vi "read Txt Files.vi"(10 "file path (use dialog)":path) -> (1 "error out":errorcluster, 2 "number":T1)   [LabVIEW 2017] (continued)
0.000000\tVoltage¡G\t4.590790\nReal Periold(ms)¡G\t1\tEncoder Position(0.1mm)¡G\t1.000000\tVelocity(0.1mm0/s)¡G\t1000.000000\tVoltage¡G\t4.606384\nReal Periold(ms)¡G\t1\tEncoder Position(0.1mm)¡G\t3.000000\tVelocity(0.1mm0/s)¡G\t2000.000000\tVoltage¡G\t4.604797\nReal Periold(ms)¡G\t1\tEncoder Position(0.1mm)¡G\t11.000000\tVelocity(0.1mm0/s)¡G\t8000.000000\tVoltage¡G\t4.602234\nReal Periold(ms)¡G\t1\tEncoder Position(0.1mm)¡G\t25.000000\tVelocity(0.1mm0/s)¡G\t14000.000000\tVoltage¡G\t4.613708\nReal Periold(ms)¡G\t1\tEncoder Position(0.1mm)¡G\t47.000000\tVelocity(0.1mm0/s)¡G\t22000.000000\tVoltage¡G\t4.615601\nReal Periold(ms)¡G\t1\tEncoder Position(0.1mm)¡G\t83.000000\tVelocity(0.1mm0/s)¡G\t36000.000000\tVoltage¡G\t4.616241\nReal Periold(ms)¡G\t1\tEncoder Position(0.1mm)¡G\t119.000000\tVelocity(0.1mm0/s)¡G\t36000.000000\tVoltage¡G\t4.597778\nReal Periold(ms)¡G\t1\tEncoder Position(0.1mm)¡G\t165.000000\tVelocity(0.1mm0/s)¡G\t46000.000000\tVoltage¡G\t4.604462\nReal Periold(ms)¡G\t1\tEncoder Position(0.1mm)¡G\t217.000000\tVelocity(0.1mm0/s)¡G\t52000.000000\tVoltage¡G\t4.609253\nReal Periold(ms)¡G\t1\tEncoder Position(0.1mm)¡G\t272.000000\tVelocity(0.1mm0/s)¡G\t55000.000000\tVoltage¡G\t4.602570\nReal Periold(ms)¡G\t1\tEncoder Position(0.1mm)¡G\t332.000000\tVelocity(0.1mm0/s)¡G\t60000.000000\tVoltage¡G\t4.608612\nReal Periold(ms)¡G\t1\tEncoder Position(0.1mm)¡G\t392.000000\tVelocity(0.1mm0/s)¡G\t60000.000000\tVoltage¡G\t4.596497\nReal Periold(ms)¡G\t1\tEncoder Position(0.1mm)¡G\t454.000000\tVelocity(0.1mm0/s)¡G\t62000.000000\tVoltage¡G\t4.605408\nReal Periold(ms)¡G\t1\tEncoder Position(0.1mm)¡G\t517.000000\tVelocity(0.1mm0/s)¡G\t63000.000000\tVoltage¡G\t4.608276\nReal Periold(ms)¡G\t1\tEncoder Position(0.1mm)¡G\t580.000000\tVelocity(0.1mm0/s)¡G\t63000.000000\tVoltage¡G\t4.619110\nReal Periold(ms)¡G\t1\tEncoder Position(0.1mm)¡G\t645.000000\tVelocity(0.1mm0/s)¡G\t65000.000000\tVoltage¡G\t4.622284\nReal Periold(ms)¡G\t1\tEncoder Position(0.1mm)¡G\t713.000000\tVelocity(0.1mm0/s)¡G\t68000.000000\tVoltage¡G\t4.615295\nReal Periold(ms)¡G\t1\tEncoder Position(0.1mm)¡G\t777.000000\tVelocity(0.1mm0/s)¡G\t64000.000000\tVoltage¡G\t4.594604\nReal Periold(ms)¡G\t1\tEncoder Position(0.1mm)¡G\t841.000000\tVelocity(0.1mm0/s)¡G\t64000.000000\tVoltage¡G\t4.611481\nReal Periold(ms)¡G\t1\tEncoder Position(0.1mm)¡G\t907.000000\tVelocity(0.1mm0/s)¡G\t66000.000000\tVoltage¡G\t4.625153\nReal Periold(ms)¡G\t1\tEncoder Position(0.1mm)¡G\t976.000000\tVelocity(0.1mm0/s)¡G\t69000.000000\tVoltage¡G\t4.610840\nReal Periold(ms)¡G\t1\tEncoder Position(0.1mm)¡G\t1038.000000\tVelocity(0.1mm0/s)¡G\t62000.000000\tVoltage¡G\t4.601929\nReal Periold(ms)¡G\t1\tEncoder Position(0.1mm)¡G\t1105.000000\tVelocity(0.1mm0/s)¡G\t67000.000000\tVoltage¡G\t4.601929\nReal Periold(ms)¡G\t1\tEncoder Position(0.1mm)¡G\t1174.000000\tVelocity(0.1mm0/s)¡G\t69000.000000\tVoltage¡G\t4.607330\nReal Periold(ms)¡G\t1\tEncoder Position(0.1mm)¡G\t1233.000000\tVelocity(0.1mm0/s)¡G\t59000.000000\tVoltage¡G\t4.600342\nReal Periold(ms)¡G\t1\tEncoder Position(0.1mm)¡G\t1303.000000\tVelocity(0.1mm0/s)¡G\t70000.000000\tVoltage¡G\t4.620697\nReal Periold(ms)¡G\t1\tEncoder Position(0.1mm)¡G\t1369.000000\tVelocity(0.1mm0/s)¡G\t66000.000000\tVoltage¡G\t4.611786\nReal Periold(ms)¡G\t1\tEncoder Position(0.1mm)¡G\t1431.000000\tVelocity(0.1mm0/s)¡G\t62000.000000\tVoltage¡G\t4.608276\nReal Periold(ms)¡G\t1\tEncoder Position(0.1mm)¡G\t1502.000000\tVelocity(0.1mm0/s)¡G\t71000.000000\tVoltage¡G\t4.606689\nReal Periold(ms)¡G\t1\tEncoder Position(0.1mm)¡G\t1564.000000\tVelocity(0.1mm0/s)¡G\t62000.000000\tVoltage¡G\t4.608276\nReal Periold(ms)¡G\t1\tEncoder Position(0.1mm)¡G\t1628.000000\tVelocity(0.1mm0/s)¡G\t64000.000000\tVoltage¡G\t4.612427\nReal Periold(ms)¡G\t1\tEncoder Position(0.1mm)¡G\t1693.000000\tVelocity(0.1mm0/s)¡G\t65000.000000\tVoltage¡G\t4.626740\nReal Periold(ms)¡G\t1\tEncoder Position(0.1mm)¡G\t1757.000000\tVelocity(0.1mm0/s)¡G\t64000.000000\tVoltage¡G\t4.596832\nReal Periold(ms)¡G\t1\tEncoder Position(0.1mm)¡G\t1823.000000\tVelocity(0.1mm0/s)¡G\t66000.000000\tVoltage¡G\t4.600006\nReal Periold(ms)¡G\t1\tEncoder Position(0.1mm)¡G\t1887.000000\tVelocity(0.1mm0/s)¡G\t64000.000000\tVoltage¡G\t4.604156\nReal Periold(ms)¡G\t1\tEncoder Position(0.1mm)¡G\t1952.000000\tVelocity(0.1mm0/s)¡G\t65000.000000\tVoltage¡G\t4.615936\nReal Periold(ms)¡G\t1\tEncoder Position(0.1mm)¡G\t2017.000000\tVelocity(0.1mm0/s)¡G\t65000.000000\tVoltage¡G\t4.612091\nReal Periold(ms)¡G\t1\tEncoder Position(0.1mm)¡G\t2079.000000\tVelocity(0.1mm0/s)¡G\t62000.000000\tVoltage¡G\t4.621979\nReal Periold(ms)¡G\t1\tEncoder Position(0.1mm)¡G\t2143.000000\tVelocity(0.1mm0/s)¡G\t64000.000000\tVoltage¡G\t4.616882\n"
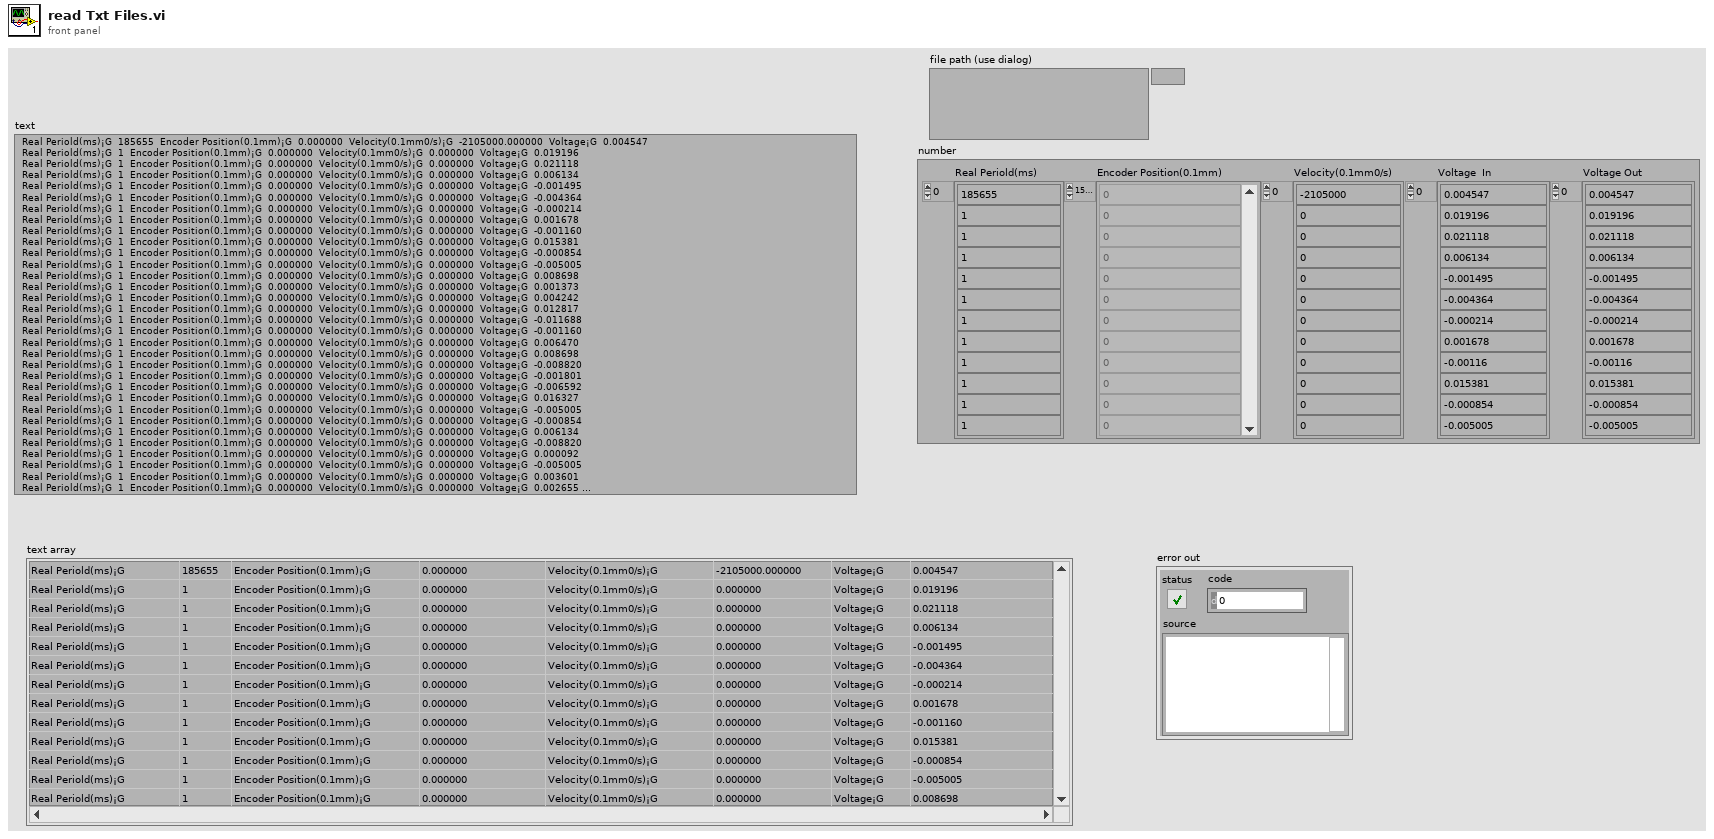
[diagram p1: front panel]
types:
  T1 = cluster{"Real Periold(ms)":dbl[], "Encoder Position(0.1mm)":dbl[], "Velocity(0.1mm0/s)":dbl[], "Voltage  In":dbl[], "Voltage Out":dbl[]}
  T2 = cluster{"Real Periold(ms)":string[], "Encoder Position(0.1mm)":string[], "Velocity(0.1mm0/s)":string[], "Voltage":string[], "Voltage 2":string[]}
  T3 = cluster{"Real Periold(ms)":dbl[], "Encoder Position(0.1mm)":dbl[], "Velocity(0.1mm0/s)":dbl[], "Voltage":dbl[], "Voltage 2":dbl[]}
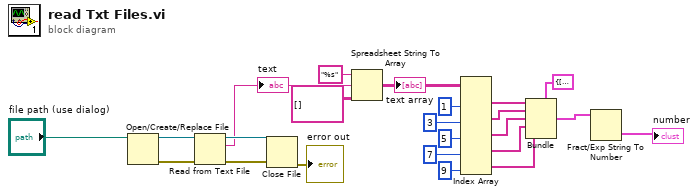
[diagram p0: block diagram]
diagram:
  n1 = Open/Create/Replace File(file path (use dialog)="file path (use dialog)") -> (refnum out=w23:refnum<file>, error out=w22:errorcluster)  [unwired: 5 in, 1 out]
  n2 = Read from Text File(file (use dialog)=w23, error in=w22) -> (refnum out=w21:refnum<file>, text=w19:string, error out=w20:errorcluster)  [unwired: 2 in, 1 out]
  "text" <- w19
  n3 = Close File(refnum=w21, error in=w20) -> (error out=→"error out":errorcluster)  [unwired: 1 out]
  n4 = Spreadsheet String To Array(format string="%s", spreadsheet string=w19, array type (2D Dbl)=string[][] []) -> (array=w16:string[][])  [unwired: 1 in]
  "text array" <- w16
  n5 = Index Array(array=w16, index (col) #1=1 ("disabled index (col)"), index (col) #2=3 ("index (col)"), index (col) #3=5 ("index (col)"), index (col) #4=7 ("index (col)"), index (col) #5=9 ("index (col)")) -> (element #1=w11:string[], element #2=w10:string[], element #3=w9:string[], element #4=w8:string[], element #5=w2:string[])  [unwired: 5 in]
  n6 = Bundle(cluster=T2 {"Real Periold(ms)"=[], "Encoder Position(0.1mm)"=[], "Velocity(0.1mm0/s)"=[], "Voltage"=[], "Voltage 2"=[]} ("number"), "Real Periold(ms)"=w11, "Encoder Position(0.1mm)"=w10, "Velocity(0.1mm0/s)"=w9, "Voltage"=w8, "Voltage 2"=w2) -> (w7:T2)
  n7 = Fract/Exp String To Number(string=w7) -> (number=→"number":T3)  [unwired: 3 in, 1 out]
